vi "Init Last Temperatures Map.vi"(8 "error in":errorcluster, 11 "Thermometer DAQmx RTD Cont CFG in":refnum<class "Thermometer DAQmx TC Cont CFG.lvclass">) -> (0 "error out":errorcluster, 3 "Thermometer DAQmx RTD Cont CFG out":refnum<class "Thermometer DAQmx TC Cont CFG.lvclass">)   [LabVIEW 2024, in "Thermometer DAQmx TC Cont CFG.lvclass"]
uses:
  Thermometer DAQmx TC Cont CFG.lvclass
  Thermometer DAQmx TC Cont CFG.lvclass/Thermometer DAQmx TC Cont CFG.ctl
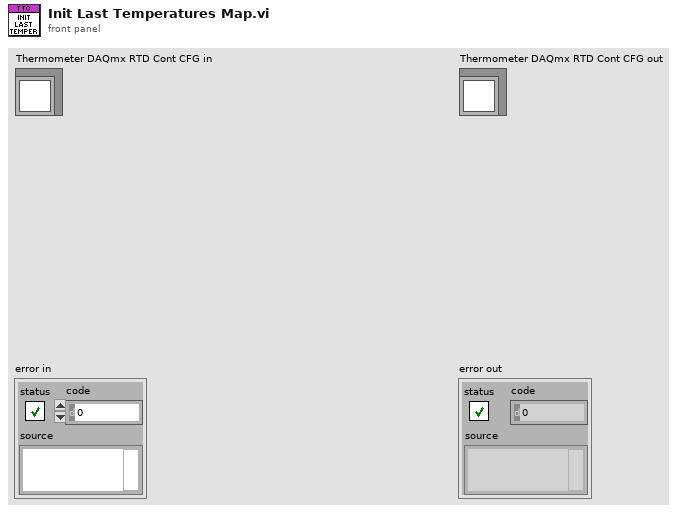
[diagram p1: front panel]
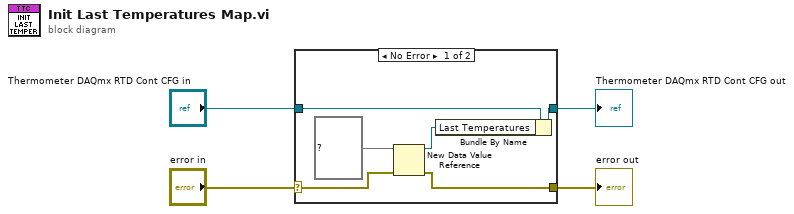
[diagram p0: block diagram]
diagram:
  n1 = case shown="No Error" "error in" {
    selector: "error in" -> [w6 w12]
    tunnel: [w5 w12] -> w3
    tunnel: [w8 w11] -> w1
    tunnel: "Thermometer DAQmx RTD Cont CFG in" -> [w10 w11]
    frame No Error {
      n2 = New Data Value Reference(data value=map{string, dbl} {} ("Temperatures"), error in=w6) -> (data value reference=w7:refnum<data-value>, error out=w5:errorcluster)
      n3 = Bundle By Name(cluster=w10, "Last Temperatures"=w7) -> (w8:refnum<class "Thermometer DAQmx TC Cont CFG.lvclass">)
    }
    frame Error {
    }
  }
  "error out" <- w3
  "Thermometer DAQmx RTD Cont CFG out" <- w1
